vi "AssertsNotEqual.vi"(11 "error in (no error)":errorcluster) -> (15 "error out":errorcluster)   [LabVIEW 2016, in "DronaTest.lvlib"]
uses:
  APIs/Assert/AssertControlValue/NotEqual.vi
  <vilib>/addons/_JKI Toolkits/Caraya/classes/Assert/Assert Not Error.vi
  <vilib>/addons/_JKI Toolkits/Caraya/classes/Assert/Assert Error.vi
  DronaTest.lvlib
  <vilib>/addons/_JKI Toolkits/Caraya/classes/Test/Test.lvclass
  Drona.lvlib
  <vilib>/addons/_JKI Toolkits/Caraya/classes/Assert/Assert.lvclass
  APIs/Assert/AssertControlValue/AssertControlValue.lvlib
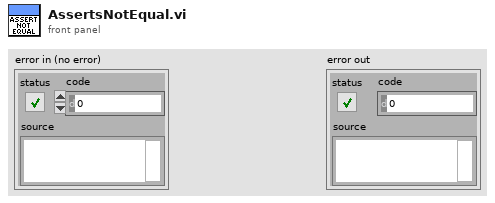
[diagram p1: front panel]
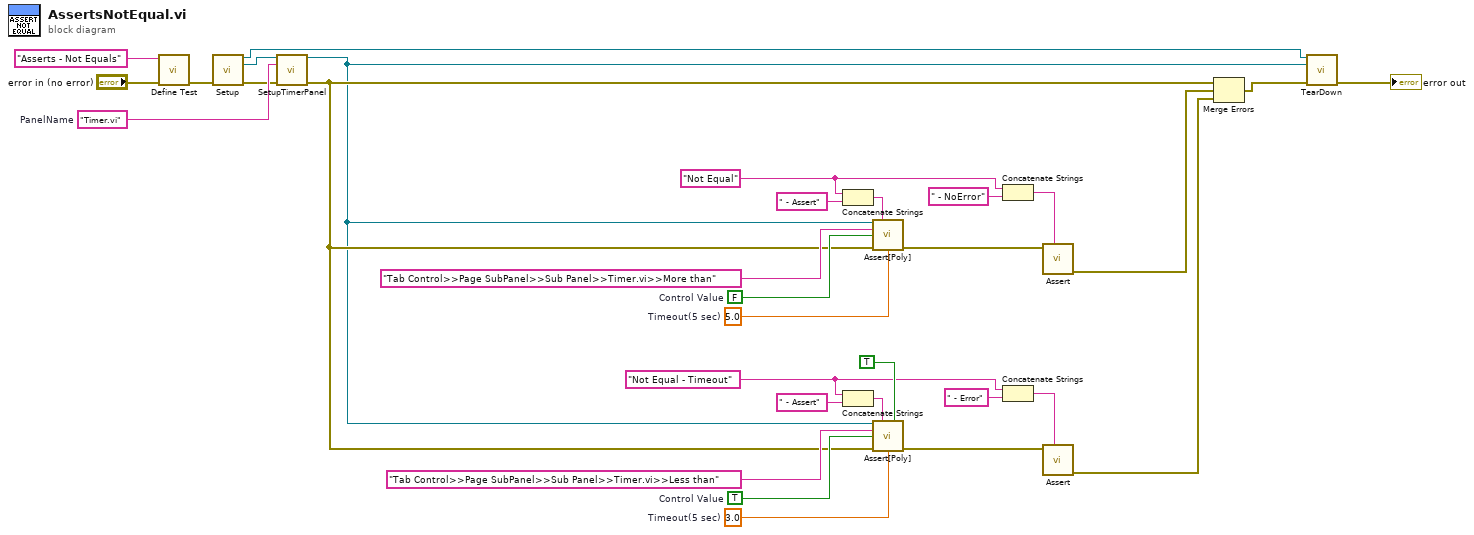
[diagram p0: block diagram]
diagram:
  w9 = "Timer.vi"  # PanelName
  w10 = TRUE  # Control Value
  w22 = 3.0  # Timeout(5 sec)
  w23 = "Not Equal - Timeout" ("string")
  w21 = 5.0  # Timeout(5 sec)
  w20 = FALSE  # Control Value
  w19 = "Not Equal" ("string")
  n1 = call <vilib>:"Define Test.vi"("error in (no error)"="error in (no error)", "Label (VI Title)"="Asserts - Not Equals") -> ("error out"=w8:errorcluster)  [unwired: 9 in]
  n2 = call "Setup.vi"("error in (no error)"=w8) -> ("Application Ref"=w5:refnum<vi>, "VI out"=w6:refnum<vi>, "error out"=w7:errorcluster)  [unwired: 12 in]
  n3 = call "SetupTimerPanel.vi"("VI in"=w6, "Panel Name"=w9, "error in (no error)"=w7) -> ("VI out"=w1:refnum<vi>, "error out"=w4:errorcluster)  [unwired: 11 in]
  n4 = Concatenate Strings(w19, " - Assert" ("string")) -> (w17:string)
  n5 = Concatenate Strings(w23, " - Assert" ("string")) -> (w25:string)
  n6 = call-poly "Assert[Poly].vi"("VI Reference In"=w1, "Test Label"=w17, "Control Path"="Tab Control>>Page SubPanel>>Sub Panel>>Timer.vi>>More than", "Control Value"=w20, "Error In"=w4, "Timeout(5 sec)"=w21) -> ("Error Out"=w16:errorcluster)  [unwired: 8 in, 1 out]
  n7 = call-poly "Assert[Poly].vi"("VI Reference In"=w1, "Test Label"=w25, "Assert Only? (F)"=TRUE, "Control Path"="Tab Control>>Page SubPanel>>Sub Panel>>Timer.vi>>Less than", "Control Value"=w10, "Error In"=w4, "Timeout(5 sec)"=w22) -> ("Error Out"=w26:errorcluster)  [unwired: 7 in, 1 out]
  n8 = Concatenate Strings(w19, " - NoError" ("string")) -> (w18:string)
  n9 = Concatenate Strings(w23, " - Error" ("string")) -> (w24:string)
  n10 = call-poly <vilib>:"Assert.vi"("Label"=w18, "Not Error?"=w16) -> ("error out"=w12:errorcluster)  [unwired: 9 in]
  n11 = call-poly <vilib>:"Assert.vi"("Label"=w24, "Error?"=w26) -> ("error out"=w11:errorcluster)  [unwired: 9 in]
  n12 = Merge Errors(w4, w12, w11) -> (w3:errorcluster)
  n13 = call "TearDown.vi"("Application Ref"=w5, "VI in"=w1, "error in (no error)"=w3) -> ("error out"=→"error out":errorcluster)  [unwired: 12 in]
